vi "KMCS2000 Initialize.vi"(8 "error in (no error)":errorcluster, 10 "timeout (10sec)":u32=10000, 11 "VISA Refnum in":refnum<visa-resource-name>) -> (0 "error out":errorcluster, 3 "VISA Refnum out":refnum<visa-resource-name>)   [LabVIEW 2018]
uses:
  <vilib>/Instr/_visa.llb/VISA Configure Serial Port (Instr).vi
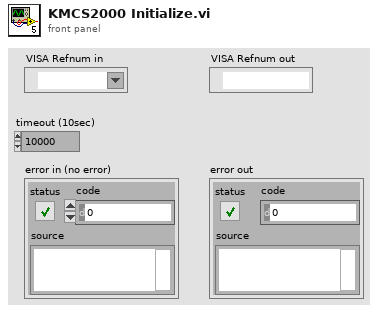
[diagram p1: front panel]
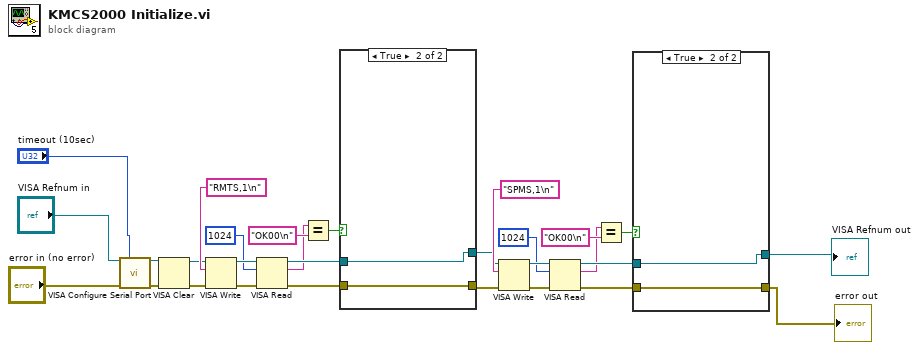
[diagram p0: block diagram]
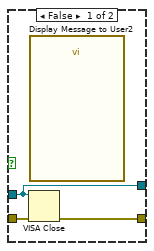
[diagram p2: hidden frame]
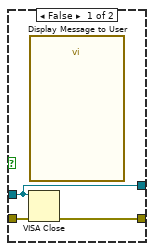
[diagram p3: hidden frame]
diagram:
  n1 = call-poly "VISA Configure Serial Port"("VISA resource name"="VISA Refnum in", "timeout (10sec)"="timeout (10sec)", "error in (no error)"="error in (no error)") -> ("VISA resource name out"=w17:refnum<visa-resource-name>, "error out"=w15:errorcluster)  [unwired: 11 in]
  n2 = VISA Clear(VISA resource name=w17, error in (no error)=w15) -> (VISA resource name out=w16:refnum<visa-resource-name>, error out=w14:errorcluster)
  n3 = VISA Write(VISA resource name=w16, write buffer="RMTS,1\n", error in (no error)=w14) -> (VISA resource name out=w21:refnum<visa-resource-name>, error out=w20:errorcluster)  [unwired: 1 out]
  n4 = VISA Read(VISA resource name=w21, byte count=u32 1024, error in (no error)=w20) -> (VISA resource name out=w28:refnum<visa-resource-name>, read buffer=w26:string, error out=w29:errorcluster)  [unwired: 1 out]
  n5 = Equal?(x=w26, y="OK00\n") -> (x = y?=w25:bool)
  n6 = case shown="True" w25 {
    tunnel: w28 -> [w30 w33]
    tunnel: w29 -> [w32 w34]
    tunnel: [w31 w34] -> w3
    tunnel: [w30 w33] -> w4
    frame False {
      n7 = VISA Close(VISA resource name=w30, error in (no error)=w32) -> (error out=w31:errorcluster)
      n8 = call "Display Message to User"() -> ()  [unwired: 10 in, 2 out]
    }
    frame True {
    }
  }
  n9 = VISA Write(VISA resource name=w4, write buffer="SPMS,1\n", error in (no error)=w3) -> (VISA resource name out=w8:refnum<visa-resource-name>, error out=w7:errorcluster)  [unwired: 1 out]
  n10 = VISA Read(VISA resource name=w8, byte count=u32 1024, error in (no error)=w7) -> (VISA resource name out=w12:refnum<visa-resource-name>, read buffer=w10:string, error out=w13:errorcluster)  [unwired: 1 out]
  n11 = Equal?(x=w10, y="OK00\n") -> (x = y?=w9:bool)
  n12 = case shown="True" w9 {
    tunnel: w12 -> [w35 w38]
    tunnel: w13 -> [w37 w39]
    tunnel: [w36 w39] -> w1
    tunnel: [w35 w38] -> w2
    frame False {
      n13 = VISA Close(VISA resource name=w35, error in (no error)=w37) -> (error out=w36:errorcluster)
      n14 = call "Display Message to User2"() -> ()  [unwired: 10 in, 2 out]
    }
    frame True {
    }
  }
  "VISA Refnum out" <- w2
  "error out" <- w1
